vi "get_data.vi"(0 "HGF_DSCService.lvclass in":refnum<class "HGF_DSCService.lvclass">, 5 "error in (no error)":errorcluster) -> (14 "HGF_DSCService.lvclass out":refnum<class "HGF_DSCService.lvclass">, 15 "serviceID":i32, 16 "data":string, 17 "quality":i32, 19 "error out":errorcluster)   [LabVIEW 2012, in "HGF_DSC.lvlib" / "HGF_DSCService.lvclass"]
uses:
  HGF_DSCService.lvclass
  HGF_DSCService.lvclass/HGF_DSCService.ctl
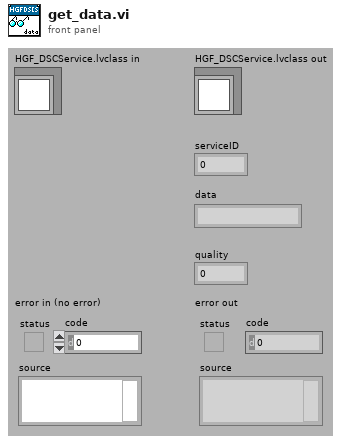
[diagram p1: front panel]
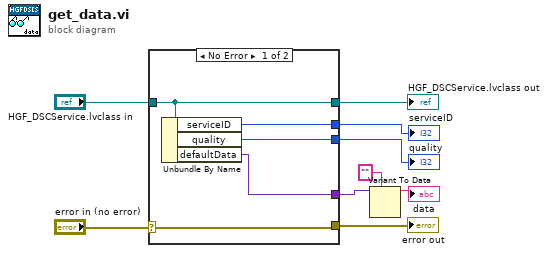
[diagram p0: block diagram]
diagram:
  n1 = case shown="No Error" "error in (no error)" {
    selector: "error in (no error)" -> [w14 w15]
    tunnel: [w14 w15] -> w8
    tunnel: "HGF_DSCService.lvclass in" -> [w13 w16]
    tunnel: [w13 w16] -> w6
    tunnel: [w12 _] -> w5
    tunnel: [w11 _] -> w4
    tunnel: [w10 _] -> w3
    frame No Error {
      n2 = Unbundle By Name(w13) -> ("serviceID"=w12:i32, "quality"=w11:i32, "defaultData"=w10:variant)
    }
    frame Error {
    }
  }
  "error out" <- w8
  "HGF_DSCService.lvclass out" <- w6
  "serviceID" <- w5
  "quality" <- w4
  n3 = Variant To Data(type="" ("data 2"), Variant=w3) -> (data=→"data":string)  [unwired: 1 in, 1 out]
